vi "Run.vi"(5 "Sequence Control":T9, 6 "Seq Name":string, 7 "VolatusAPI":refnum<class "VolatusAPI.lvclass">, 10 "State Loop Data in":T1, 11 "State in":refnum<class "State.lvclass">) -> (2 "State Loop Data":T1, 3 "State out":refnum<class "State.lvclass">)   [LabVIEW 2023, in "VolatusSeq.lvlib" / "State.lvclass"]
uses:
  State.lvclass
  Volatus/VolatusAPI/VolatusAPI.lvclass
  State Loop Data.ctl
  Iteration Actions/Iteration Actions.lvclass
  Variables/Variables.lvclass
  Command.ctl
  Volatus/MessageQ/MessageQ.lvclass
  Format String/Format String.lvclass
  VolatusSeqConfig/Command Type.ctl
  messages/CmdDigital/Data.ctl
  messages/CmdAnalog/Data.ctl
  Send Type.ctl
  lv-vecto/Vecto/Channel DBL/Channel DBL.lvclass
  Transition/Transition.lvclass
  Sequence Time.ctl
  VolatusSeqConfig/Debug Flags.ctl
  State Control.ctl
  State.lvclass/State.ctl
  Volatus/VolatusAPI/Report Event.vi
  VolatusSeq.lvlib
  VolatusSeqConfig/VolatusSeqConfig.lvlib
  messages/CmdDigital/CmdDigital.lvlib
  messages/CmdAnalog/CmdAnalog.lvlib
panel:
  out "Live State":T1
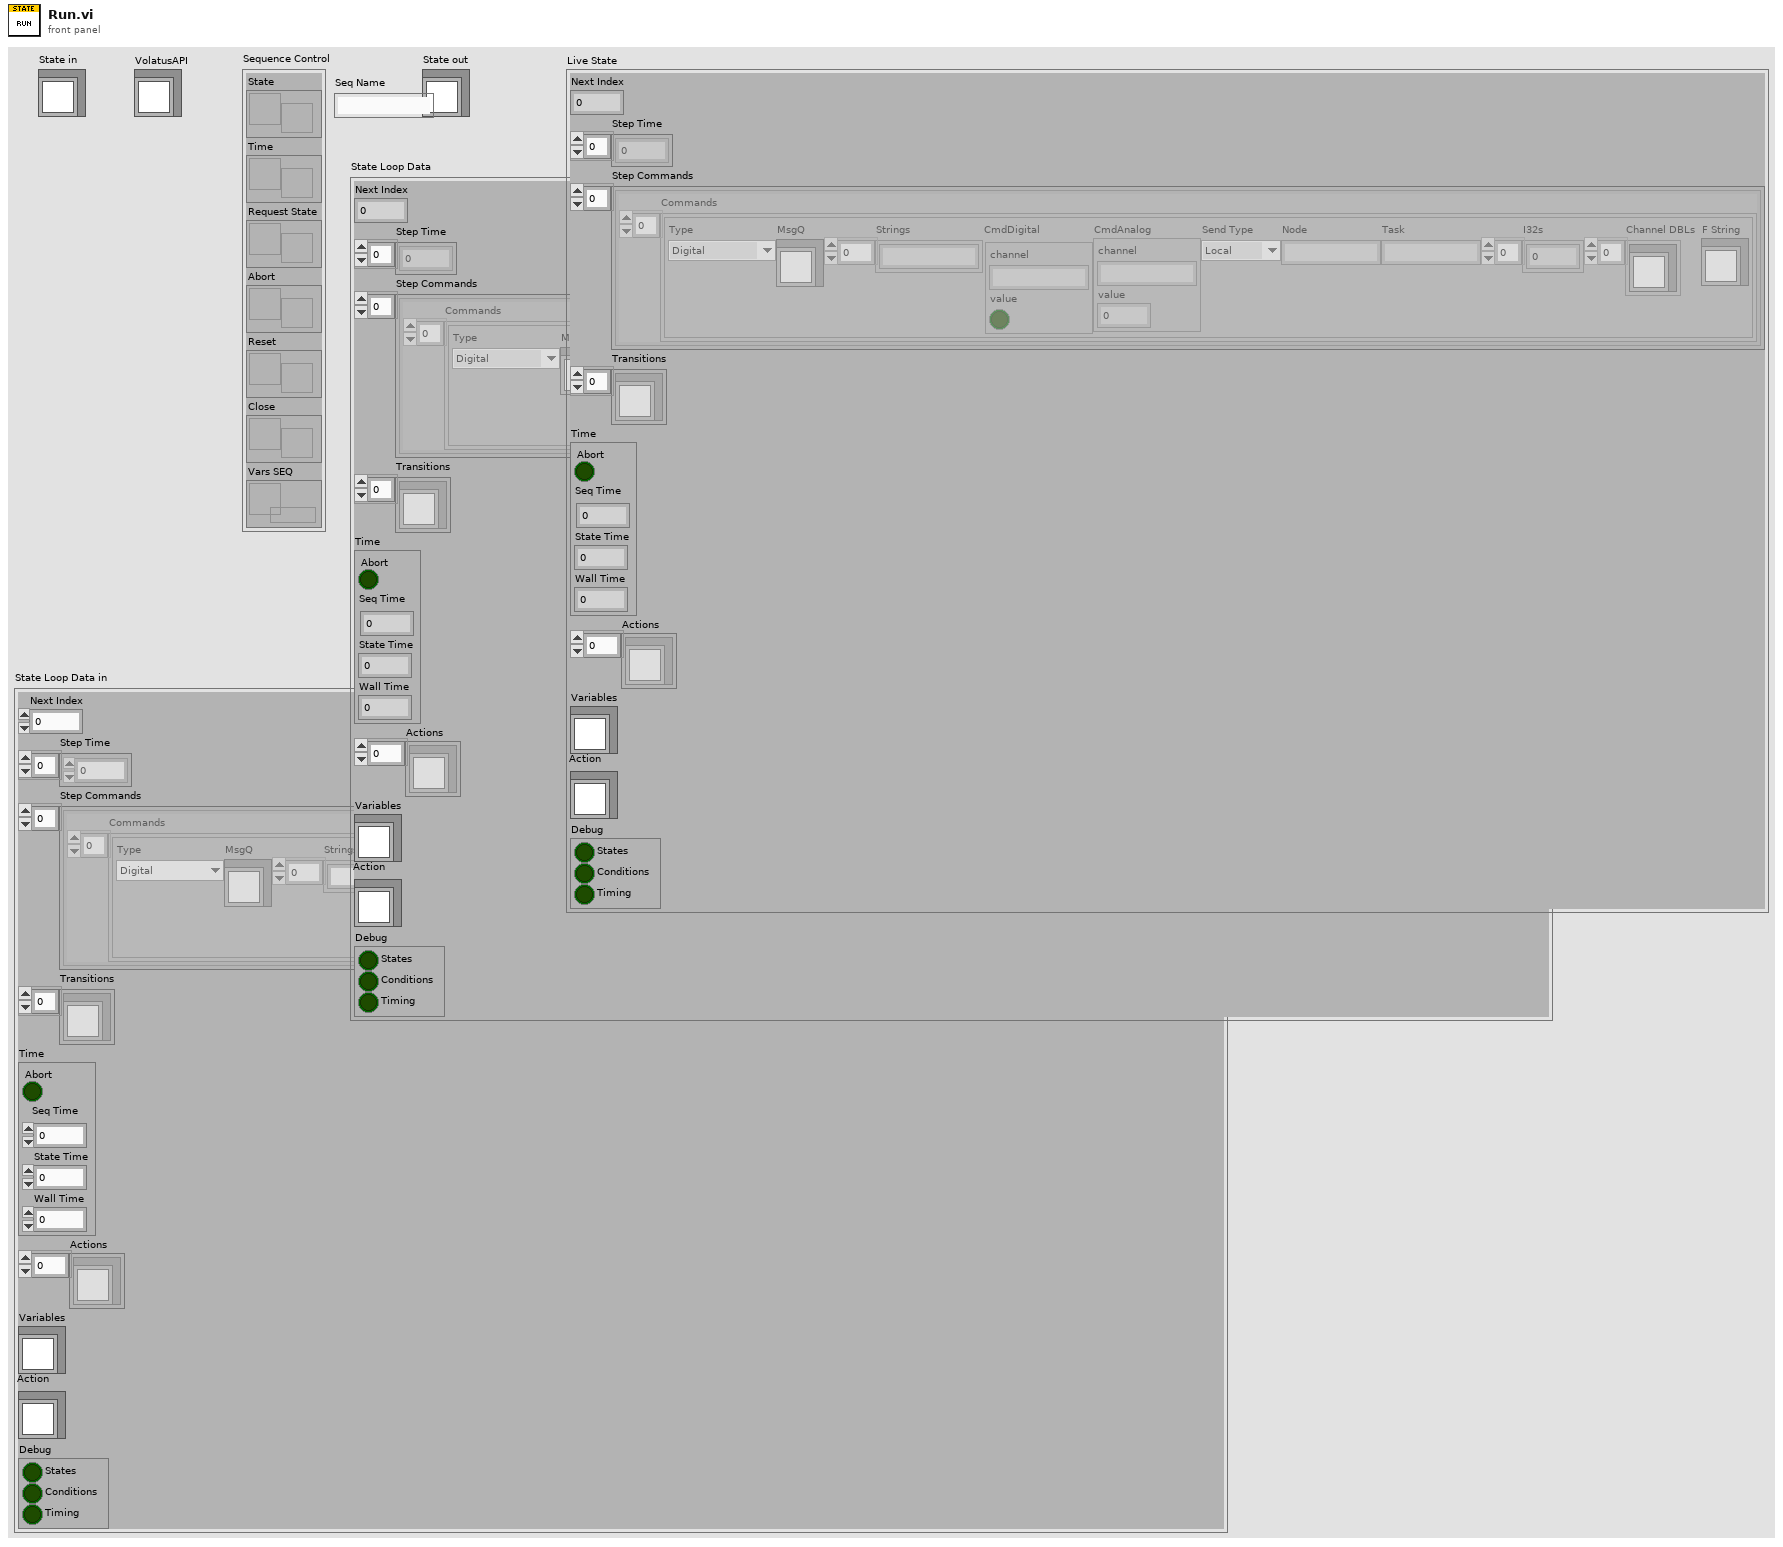
[diagram p1: front panel]
types:
  T1 = typedef "VolatusSeq.lvlib/State.lvclass/State Loop Data.ctl" = cluster{"Next Index":i32, "Step Time":dbl[], "Step Commands":cluster{"Commands":T2[]}[], "Transitions":refnum<class "Transition.lvclass">[], "Time":T7, "Actions":refnum<class "Iteration Actions.lvclass">[], "Variables":refnum<class "Variables.lvclass">, "Action":refnum<class "Iteration Actions.lvclass">, "Debug":T8}
  T2 = typedef "VolatusSeq.lvlib/Command.ctl" = cluster{"Type":T3, "MsgQ":refnum<class "MessageQ.lvclass">, "Strings":string[], "CmdDigital":T4, "CmdAnalog":T5, "Send Type":T6, "Node":string, "Task":string, "I32s":i32[], "Channel DBLs":refnum<class "Channel DBL.lvclass">[], "F String":refnum<class "Format String.lvclass">}
  T3 = typedef "VolatusSeqConfig.lvlib/Command Type.ctl" = enum16{"Digital", "Numeric", "Transition", "Stop", "StartLog", "StopLog", "Start", "Event", "Error", "HTTP", "ResetVar", "IncVar", "DecVar", "SaveVar", "LoadVar", "AddVar", "SubVar", "SetVar", "AddToVar"}
  T4 = typedef "CmdDigital.lvlib/Data.ctl" = cluster{"channel":string, "value":bool}
  T5 = typedef "CmdAnalog.lvlib/Data.ctl" = cluster{"channel":string, "value":dbl}
  T6 = typedef "VolatusSeq.lvlib/Send Type.ctl" = enum16{"Local", "Remote"}
  T7 = typedef "VolatusSeq.lvlib/Sequence Time.ctl" = cluster{"Abort":bool, "Seq Time":dbl, "State Time":dbl, "Wall Time":dbl}
  T8 = typedef "VolatusSeqConfig.lvlib/Debug Flags.ctl" = cluster{"States":bool, "Conditions":bool, "Timing":bool}
  T9 = typedef "VolatusSeq.lvlib/State Control.ctl" = cluster{"State":refnum<notifier>, "Time":refnum<notifier>, "Request State":refnum<notifier>, "Abort":refnum<notifier>, "Reset":refnum<notifier>, "Close":refnum<notifier>, "Vars SEQ":refnum<queue>}
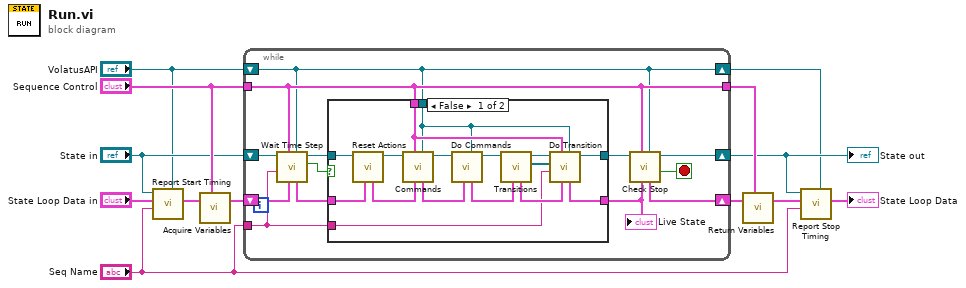
[diagram p0: block diagram]
diagram:
  n1 = call "Report Start Timing.vi"("VolatusAPI"="VolatusAPI", "Seq Name"="Seq Name", "State Loop Data In"="State Loop Data in", "State in"="State in") -> ("State Loop Data"=w8:T1)  [unwired: 7 in]
  n2 = call "Acquire Variables.vi"("State Loop Data In"=w8, "State Control"="Sequence Control") -> ("State Loop Data"=w11:T1)  [unwired: 5 in]
  n3 = while {
    shift-right: [w21] -> w3
    shift-left: "State in" -> [w17]
    tunnel: "Sequence Control" -> [w16]
    shift-right: [w19] -> w12
    shift-left: w11 -> [w23]
    tunnel: "Seq Name" -> [w15]
    tunnel: [w16] -> w9
    shift-right: [w14] -> w2
    shift-left: "VolatusAPI" -> [w14]
    stop <- w18 stop-if-true
    n4 = call "Wait Time Step.vi"("VolatusAPI"=w14, "State Loop Data in"=w23, "State Control"=w16, "Seq Name"=w15, "State in"=w17) -> ("Abort"=w24:bool, "State out"=w26:refnum<class "State.lvclass">, "State Loop Data"=w25:T1)  [unwired: 4 in]
    n5 = case shown="False" w24 {
      tunnel: w26 -> [w42 w44]
      tunnel: w16 -> [w33 _]
      tunnel: w14 -> [w32 _]
      tunnel: w25 -> [w27 w43]
      tunnel: [w34 w43] -> w20
      tunnel: [w36 w44] -> w22
      tunnel: w15 -> [w31 _]
      frame False {
        n6 = call "Reset Actions.vi"("State Loop Data in"=w27, "State in"=w42) -> ("State out"=w29:refnum<class "State.lvclass">, "State Loop Data"=w28:T1)  [unwired: 8 in]
        n7 = call "Commands.vi"("VolatusAPI"=w32, "State Loop Data in"=w28, "State Control"=w33, "State in"=w29) -> ("State out"=w41:refnum<class "State.lvclass">, "State Loop Data"=w38:T1)  [unwired: 6 in]
        n8 = call "Do Commands.vi"("VolatusAPI"=w32, "State Loop Data in"=w38, "State in"=w41) -> ("State out"=w39:refnum<class "State.lvclass">, "State Loop Data"=w37:T1)  [unwired: 7 in]
        n9 = call "Transitions.vi"("State Loop Data in"=w37, "State in"=w39) -> ("Met Conditions"=w30:refnum<class "Condition.lvclass">[], "State out"=w40:refnum<class "State.lvclass">, "State Loop Data"=w35:T1)  [unwired: 7 in]
        n10 = call "Do Transition.vi"("VolatusAPI"=w32, "State Loop Data in"=w35, "State Control"=w33, "Seq Name"=w31, "Met Conditions"=w30, "State in"=w40) -> ("State out"=w36:refnum<class "State.lvclass">, "State Loop Data"=w34:T1)  [unwired: 4 in]
      }
      frame True {
      }
    }
    "Live State" <- w20
    n11 = call "Check Stop.vi"("VolatusAPI"=w14, "State Loop Data in"=w20, "State Control"=w16, "State in"=w22) -> ("Stop"=w18:bool, "State out"=w21:refnum<class "State.lvclass">, "State Loop Data"=w19:T1)  [unwired: 5 in]
  }
  "State out" <- w3
  n12 = call "Return Variables.vi"("State Loop Data In"=w12, "State Control"=w9) -> ("State Loop Data"=w10:T1)  [unwired: 5 in]
  n13 = call "Report Stop Timing.vi"("VolatusAPI"=w2, "Seq Name"="Seq Name", "State Loop Data In"=w10, "State in"=w3) -> ("State Loop Data"=→"State Loop Data":T1)  [unwired: 7 in]
